vi "Method.vi"(4 "Value":refnum<class "Abs_U32 Integer.lvclass">) -> (1 "Result":refnum<class "Abs_U32 Integer.lvclass">)   [LabVIEW 2021, in "Decrement_U32.lvclass"]
uses:
  Decrement_U32.lvclass
  Abs_Types/U32 Integer/Abs_U32 Integer.lvclass
  C:/TSA/LV_Abstract/Source/Functions/Support/Function/One Terminal/U32/AbsFunc_One Term_U32.lvclass
  C:/Program Files (x86)/National Instruments/LabVIEW 2021/vi.lib/TSA/Abstract Data Classes/Abs_Types/U32 Integer/Abs_U32 Integer.lvclass
  Support/Function/One Terminal/U32/AbsFunc_One Term_U32.lvclass/AbsFunc_One Term_U32.ctl
  Support/Function/One Terminal/U32/Properties/Write Numeric A.vi
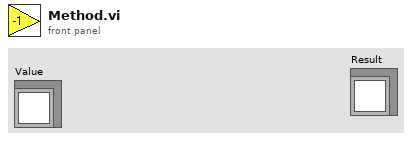
[diagram p1: front panel]
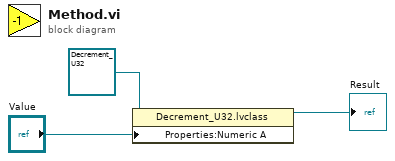
[diagram p0: block diagram]
diagram:
  n1 = property class="Decrement_U32.lvclass"(reference=refnum<class "Decrement_U32.lvclass"> refnum ("Decrement_DBL.lvclass"), "Properties:Numeric A"="Value") -> (reference out=→"Result":refnum<class "Decrement_U32.lvclass">)  [unwired: 1 in, 1 out]
